vi "Conductor.vi"(8 "entrée d'erreur (pas d'erreur)":errorcluster, 9 "Files d'attente de messages en entrée":T4, 10 "Ce VI":refnum<vi>, 11 "File d'attente en entrée":refnum<queue>) -> (0 "sortie d'erreur":T1, 2 "Data Cluster":T2, 3 "File d'attente en sortie":refnum<queue>)   [LabVIEW 2020]
uses:
  support/Message Queue/All Message Queues.ctl
  support/Message Queue/Message Cluster.ctl
  controls/UI Data.ctl
  controls/Ctrl_display.ctl
  support/Message Queue/Enqueue Message (Single).vi
  <vilib>/Utility/error.llb/Error Cluster From Error Code.vi
  <vilib>/ErrorRing/Error Ring.xnode
  support/Message Queue/Message Queue.lvlib
  support/User Event - Stop/User Event - Stop.lvlib
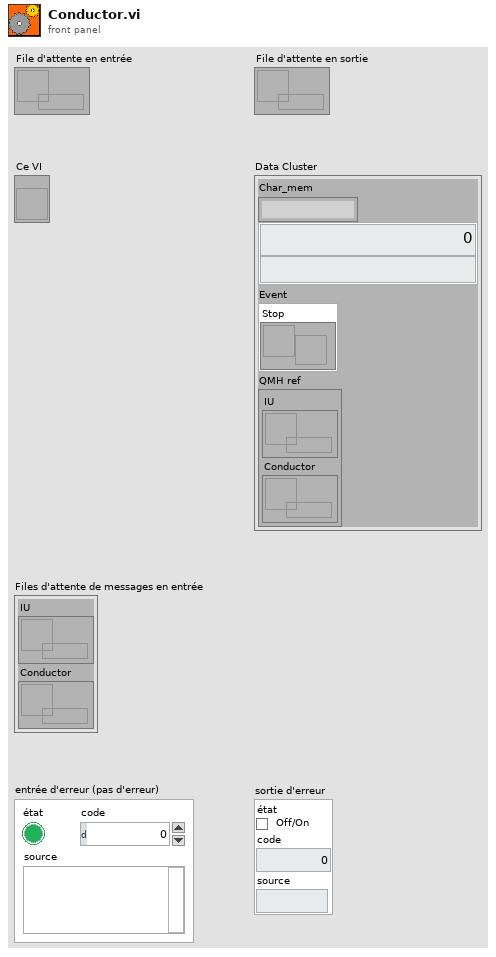
[diagram p1: front panel]
types:
  T1 = cluster{"état":bool, "code":i32, "source":string}
  T2 = typedef "UI Data.ctl" = cluster{"Char_mem":string, "Display":T3, "Event":cluster{"Stop":refnum<user-event>}, "QMH ref":T4}
  T3 = typedef "Ctrl_display.ctl" = cluster{"Num":dbl, "Char":string}
  T4 = typedef "Message Queue.lvlib/All Message Queues.ctl" = cluster{"IU":refnum<queue>, "Conductor":refnum<queue>}
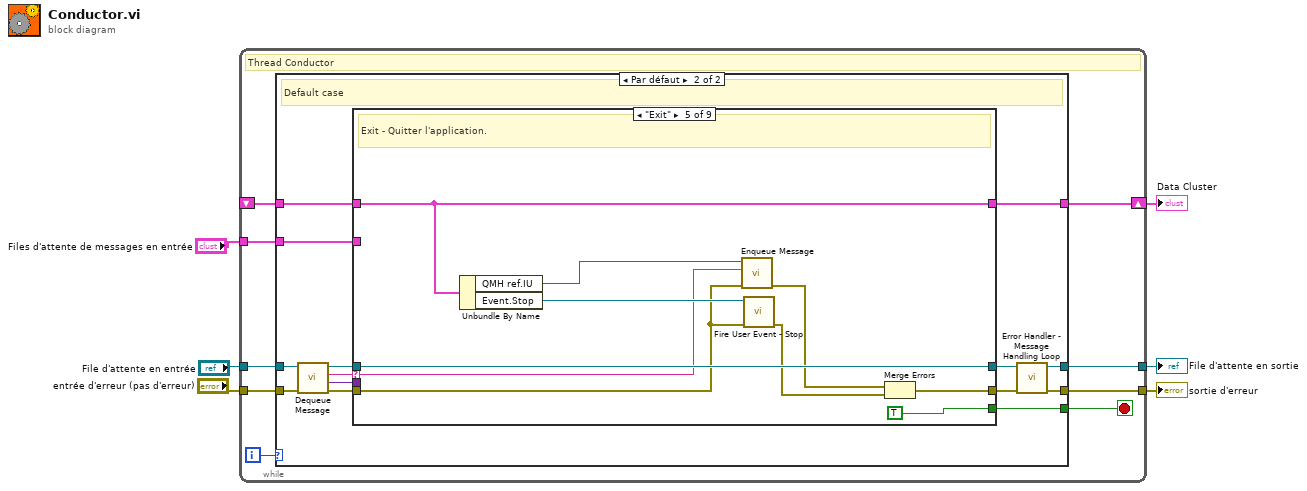
[diagram p0: block diagram]
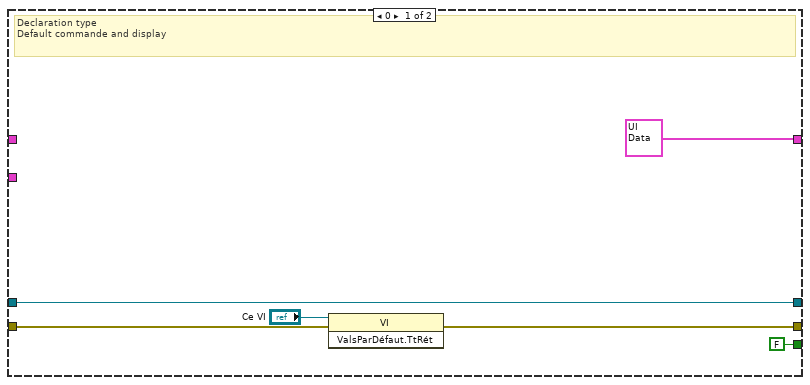
[diagram p2: hidden frame]
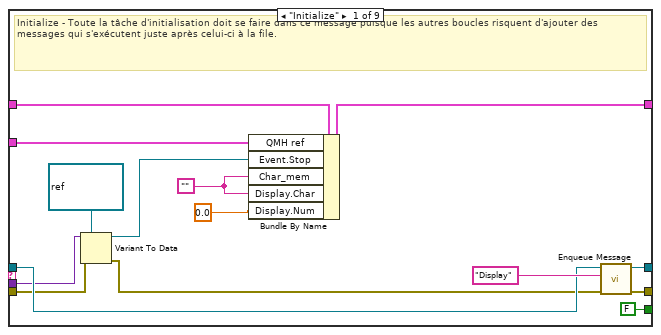
[diagram p3: hidden frame]
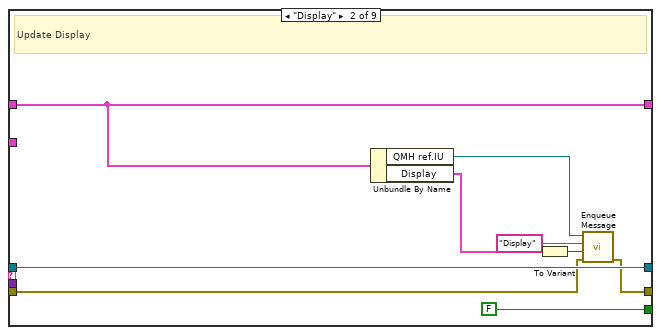
[diagram p4: hidden frame]
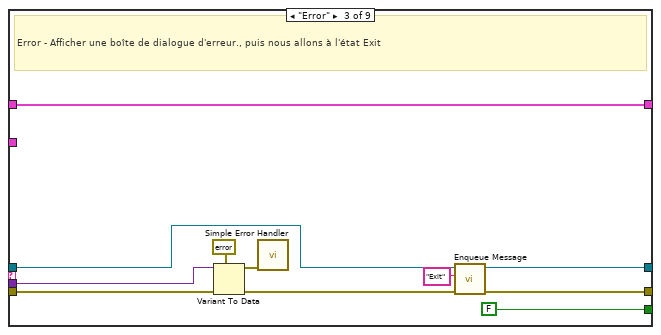
[diagram p5: hidden frame]
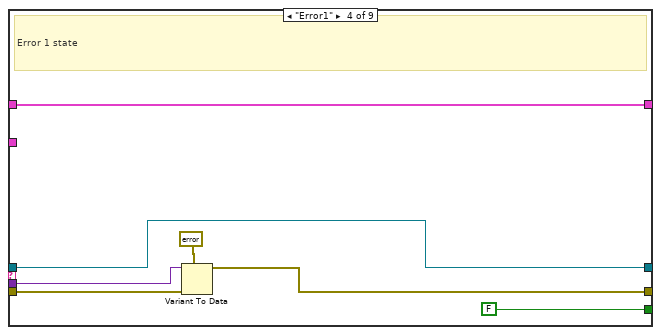
[diagram p6: hidden frame]
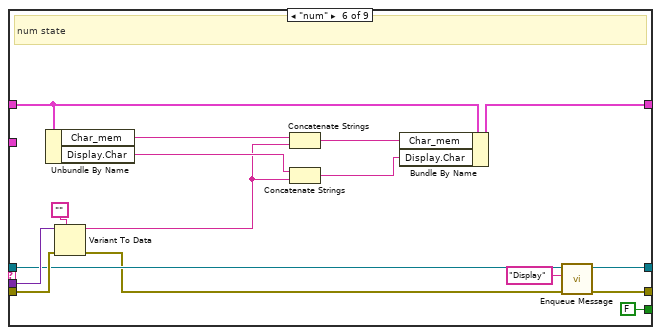
[diagram p7: hidden frame]
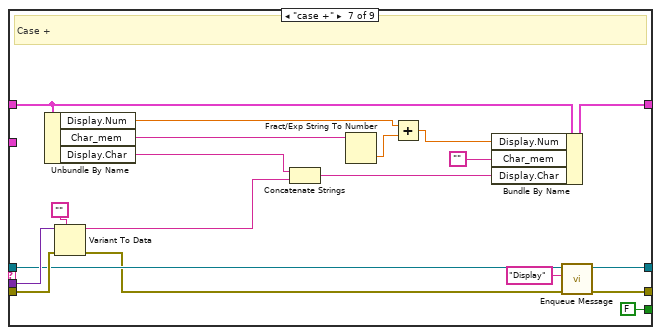
[diagram p8: hidden frame]
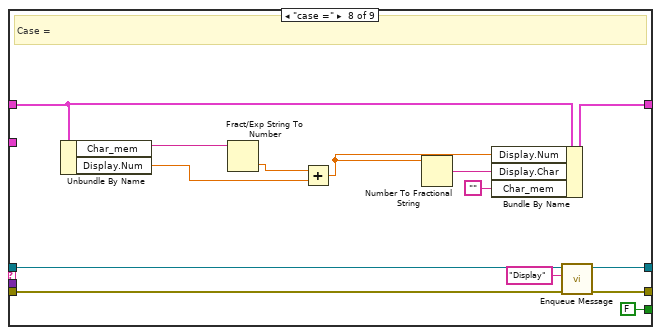
[diagram p9: hidden frame]
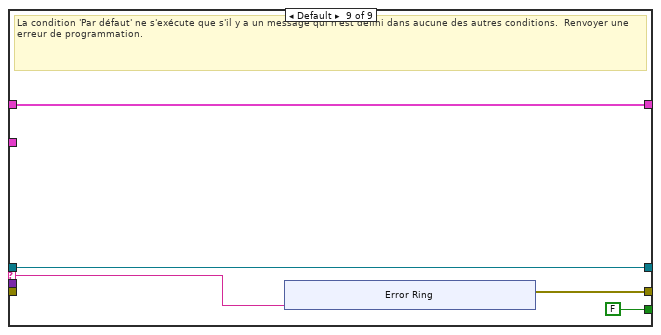
[diagram p10: hidden frame]
diagram:
  n1 = while {
    tunnel: "File d'attente en entrée" -> [w11]
    shift-right: [w14] -> w4
    shift-left: _ -> [w15]
    tunnel: "entrée d'erreur (pas d'erreur)" -> [w12]
    tunnel: [w10] -> w2
    tunnel: [w9] -> w3
    tunnel: "Files d'attente de messages en entrée" -> [w7]
    i -> [w8]
    stop <- w13 stop-if-true
    # "Thread Conductor"
    n2 = case shown="Par défaut" w8 {
      tunnel: w15 -> [_ w35]
      tunnel: [T2 {"Char_mem"="", "Display"={"Num"=0.0, "Char"=""}, "Event"={"Stop"=refnum}, "QMH ref"={"IU"=refnum, "Conductor"=refnum}} ("Data Cluster") w34] -> w14
      tunnel: [FALSE w33] -> w13
      tunnel: w12 -> [w17 w32]
      tunnel: w11 -> [w20 w28]
      tunnel: [w16 w26] -> w10
      tunnel: [w20 w23] -> w9
      tunnel: w7 -> [_ w22]
      frame 0 {
        # "Declaration type\nDefault commande and display"
        n3 = invoke class="VI" method="ValsParDéfaut.TtRét"(reference="Ce VI", error in=w17) -> (error out=w16:errorcluster)  [unwired: 1 in, 2 out]
      }
      frame Default {
        # "Default case"
        n4 = call "Dequeue Message.vi"("error in (no error)"=w32, "File d'attente de messages"=w28) -> ("error out"=w31:T1, "Données de message"=w29:variant, "Message"=w30:string, "File d'attente de message dup."=w27:refnum<queue>)  [unwired: 6 in]
        n5 = case "Conditions des messages" shown="\"Exit\"" w30 {
          selector: w30 -> [_ _ _ _ w78 _ _ _ w139]
          tunnel: w27 -> [w46 w59 w61 w71 w86 w93 w114 w134 w138]
          tunnel: w31 -> [w42 w53 w70 w77 w82 w101 w120 w129 _]
          tunnel: [w50 w52 w62 w73 w80 w91 w112 w132 w140] -> w25
          tunnel: w35 -> [w49 w55 w69 w76 w84 w100 w119 w136 w141]
          tunnel: [w48 w55 w69 w76 w84 w96 w116 w135 w141] -> w34
          tunnel: [FALSE FALSE FALSE FALSE TRUE FALSE FALSE FALSE FALSE] -> w33
          tunnel: w29 -> [w43 _ w68 w75 _ w103 w122 _ _]
          tunnel: [w45 w59 w60 w71 w86 w92 w113 w133 w138] -> w24
          tunnel: w22 -> [w36 _ _ _ _ _ _ _ _]
          frame "Initialize" {
            w38 = ""
            # "Initialize - Toute la tâche d'initialisation doit se faire dans ce message puisque les autres boucles risquent d'ajouter des messages qui s'exécutent juste après celui-ci à la file."
            n6 = Variant To Data(error in=w42, type=refnum<user-event> refnum ("Événement utilisateur - Arrêt"), Variant=w43) -> (data=w40:refnum<user-event>, error out=w39:errorcluster)
            n7 = Bundle By Name(cluster=w49, "QMH ref"=w36, "Event.Stop"=w40, "Char_mem"=w38, "Display.Char"=w38, "Display.Num"=0.0) -> (w48:T2)
            n8 = call-poly "Enqueue Message.vi"("error in (no error)"=w39, "Message"="Display", "File d'attente de messages"=w46) -> ("error out"=w50:T1, "File d'attente de message dup."=w45:refnum<queue>)  [unwired: 7 in]
          }
          frame "Display" {
            # "Update Display"
            n9 = Unbundle By Name(w55) -> ("QMH ref.IU"=w56:refnum<queue>, "Display"=w54:T3)
            n10 = To Variant(anything=w54) -> (Variant=w51:variant)
            n11 = call-poly "Enqueue Message.vi"("error in (no error)"=w53, "Données de message"=w51, "Message"="Display", "File d'attente de messages"=w56) -> ("error out"=w52:T1)  [unwired: 6 in, 1 out]
          }
          frame "Error" {
            # "Error - Afficher une boîte de dialogue d'erreur., puis nous allons à l'état Exit"
            n12 = Variant To Data(error in=w70, type=errorcluster {"status"=FALSE, "code"=0, "source"=""} ("error constant"), Variant=w68) -> (data=w66:errorcluster, error out=w63:errorcluster)
            n13 = call <vilib>:"Simple Error Handler.vi"("error in (no error)"=w66) -> ()  [unwired: 4 in, 5 out]
            n14 = call-poly "Enqueue Message.vi"("error in (no error)"=w63, "Message"="Exit", "File d'attente de messages"=w61) -> ("error out"=w62:T1, "File d'attente de message dup."=w60:refnum<queue>)  [unwired: 7 in]
          }
          frame "Error1" {
            # "Error 1 state"
            n15 = Variant To Data(error in=w77, type=errorcluster {"status"=FALSE, "code"=0, "source"=""} ("error constant"), Variant=w75) -> (data=w73:errorcluster)  [unwired: 1 out]
          }
          frame "Exit" {
            # "Exit - Quitter l'application."
            n16 = Unbundle By Name(w84) -> ("QMH ref.IU"=w81:refnum<queue>, "Event.Stop"=w83:refnum<user-event>)
            n17 = call-poly "Enqueue Message.vi"("error in (no error)"=w82, "Message"=w78, "File d'attente de messages"=w81) -> ("error out"=w79:T1)  [unwired: 7 in, 1 out]
            n18 = call "Fire User Event - Stop.vi"("error in (no error)"=w82, "Événement utilisateur - Arrêt"=w83) -> ("error out"=w85:T1)  [unwired: 9 in]
            n19 = Merge Errors(w79, w85) -> (w80:errorcluster)
          }
          frame "num" {
            # "num state"
            n20 = Unbundle By Name(w100) -> ("Char_mem"=w99:string, "Display.Char"=w98:string)
            n21 = Variant To Data(error in=w101, type="", Variant=w103) -> (data=w97:string, error out=w89:errorcluster)
            n22 = Concatenate Strings(w99, w97) -> (w95:string)
            n23 = Concatenate Strings(w98, w97) -> (w94:string)
            n24 = Bundle By Name(cluster=w100, "Char_mem"=w95, "Display.Char"=w94) -> (w96:T2)
            n25 = call-poly "Enqueue Message.vi"("error in (no error)"=w89, "Message"="Display", "File d'attente de messages"=w93) -> ("error out"=w91:T1, "File d'attente de message dup."=w92:refnum<queue>)  [unwired: 7 in]
          }
          frame "case +" {
            # "Case +"
            n26 = Unbundle By Name(w119) -> ("Display.Num"=w105:dbl, "Char_mem"=w107:string, "Display.Char"=w118:string)
            n27 = Variant To Data(error in=w120, type="", Variant=w122) -> (data=w117:string, error out=w110:errorcluster)
            n28 = Concatenate Strings(w118, w117) -> (w115:string)
            n29 = Fract/Exp String To Number(string=w107) -> (number=w106:dbl)  [unwired: 3 in, 1 out]
            n30 = Add(x=w105, y=w106) -> (x+y=w104:dbl)
            n31 = Bundle By Name(cluster=w119, "Display.Num"=w104, "Char_mem"="", "Display.Char"=w115) -> (w116:T2)
            n32 = call-poly "Enqueue Message.vi"("error in (no error)"=w110, "Message"="Display", "File d'attente de messages"=w114) -> ("error out"=w112:T1, "File d'attente de message dup."=w113:refnum<queue>)  [unwired: 7 in]
          }
          frame "case =" {
            # "Case ="
            n33 = Unbundle By Name(w136) -> ("Char_mem"=w127:string, "Display.Num"=w126:dbl)
            n34 = Fract/Exp String To Number(string=w127) -> (number=w125:dbl)  [unwired: 3 in, 1 out]
            n35 = Add(x=w125, y=w126) -> (x+y=w123:dbl)
            n36 = Number To Fractional String(number=w123) -> (F-format string=w128:string)  [unwired: 3 in]
            n37 = Bundle By Name(cluster=w136, "Display.Num"=w123, "Display.Char"=w128, "Char_mem"="") -> (w135:T2)
            n38 = call-poly "Enqueue Message.vi"("error in (no error)"=w129, "Message"="Display", "File d'attente de messages"=w134) -> ("error out"=w132:T1, "File d'attente de message dup."=w133:refnum<queue>)  [unwired: 7 in]
          }
          frame Default {
            # "La condition 'Par défaut' ne s'exécute que s'il y a un message qui n'est défini dans aucune des autres conditions.  Renvoyer une erreur de programmation."
            n39 = xnode ("Error Ring")("paramètre 0"=w139) -> ("sortie d'erreur"=w140:errorcluster)
          }
        }
        n40 = call "Error Handler - Message Handling Loop.vi"("error in (no error)"=w25, "File d'attente de messages"=w24) -> ("erreur en entrée dup."=w26:T1, "File d'attente de message dup."=w23:refnum<queue>)  [unwired: 8 in]
      }
    }
  }
  "Data Cluster" <- w4
  "File d'attente en sortie" <- w3
  "sortie d'erreur" <- w2
